vi "LabVIEW_ArduinoControls.vi"() -> ()   [LabVIEW 2020]
uses:
  <vilib>/Instr/_visa.llb/VISA Configure Serial Port (Instr).vi
panel:
  in  "DRILL STOP":bool
  in  "Drill Speed Arduino 2 Write Stop":bool
  in  "Slow Down":bool
  in  "Speed Up":bool
  in  "Drill Speed Arduino 2 Write":refnum<visa-resource-name>
  in  "Stepper Arduino 1 Serial Read":refnum<visa-resource-name>
  out "Weight on Bit A1":dbl[](graph)
  out "Vertical Motor Speed A1":dbl[](graph)
  out "Data Packet Arduini 1 Matched":i32
  in  "Arduino 1 Read Stop 2":bool
  in  "Arduino 1 Read Stop":bool
  in  "Emergency Stop! 3":bool
  in  "Emergency Stop! 2":bool
  in  "GO DOWN 3":bool
  in  "GO DOWN 2":bool
  in  "GO UP 3":bool
  in  "GO UP 2":bool
  in  "MAX SPEED 3":bool
  in  "MAX SPEED 2":bool
  in  "SLOWEST SPEED 3":bool
  in  "SLOWEST SPEED 2":bool
  in  "Decellerate 3":bool
  in  "Decellerate 2":bool
  in  "Accelerate 3":bool
  in  "Accelerate 2":bool
  in  "Drill Speed Arduino 2 Serial Read":refnum<visa-resource-name>
  out "Data Packet Received":i32
  out "Drill Amps A2":dbl[](graph)
  in  "GO UP":bool
  in  "GO DOWN":bool
  in  "MAX SPEED":bool
  in  "SLOWEST SPEED":bool
  out "System Amps A2":dbl[](graph)
  out "concatenated string":string
  in  "Arduino 2 Write Stop":bool
  in  "Emergency Stop!":bool
  in  "Decellerate":bool
  in  "Stepper Arduino 1 Write":refnum<visa-resource-name>
  in  "Accelerate":bool
  # "WINCH CONTROLS"
  # "VERTICAL STEPPER MOTOR CONTROLS"
  # "HORIZONTAL STEPPER MOTOR CONTROLS"
  # "Drill Speed Controls"
  # "-1 Means Not Found\nany value greater than 0 corresponds to the amount\nof matching characters found"
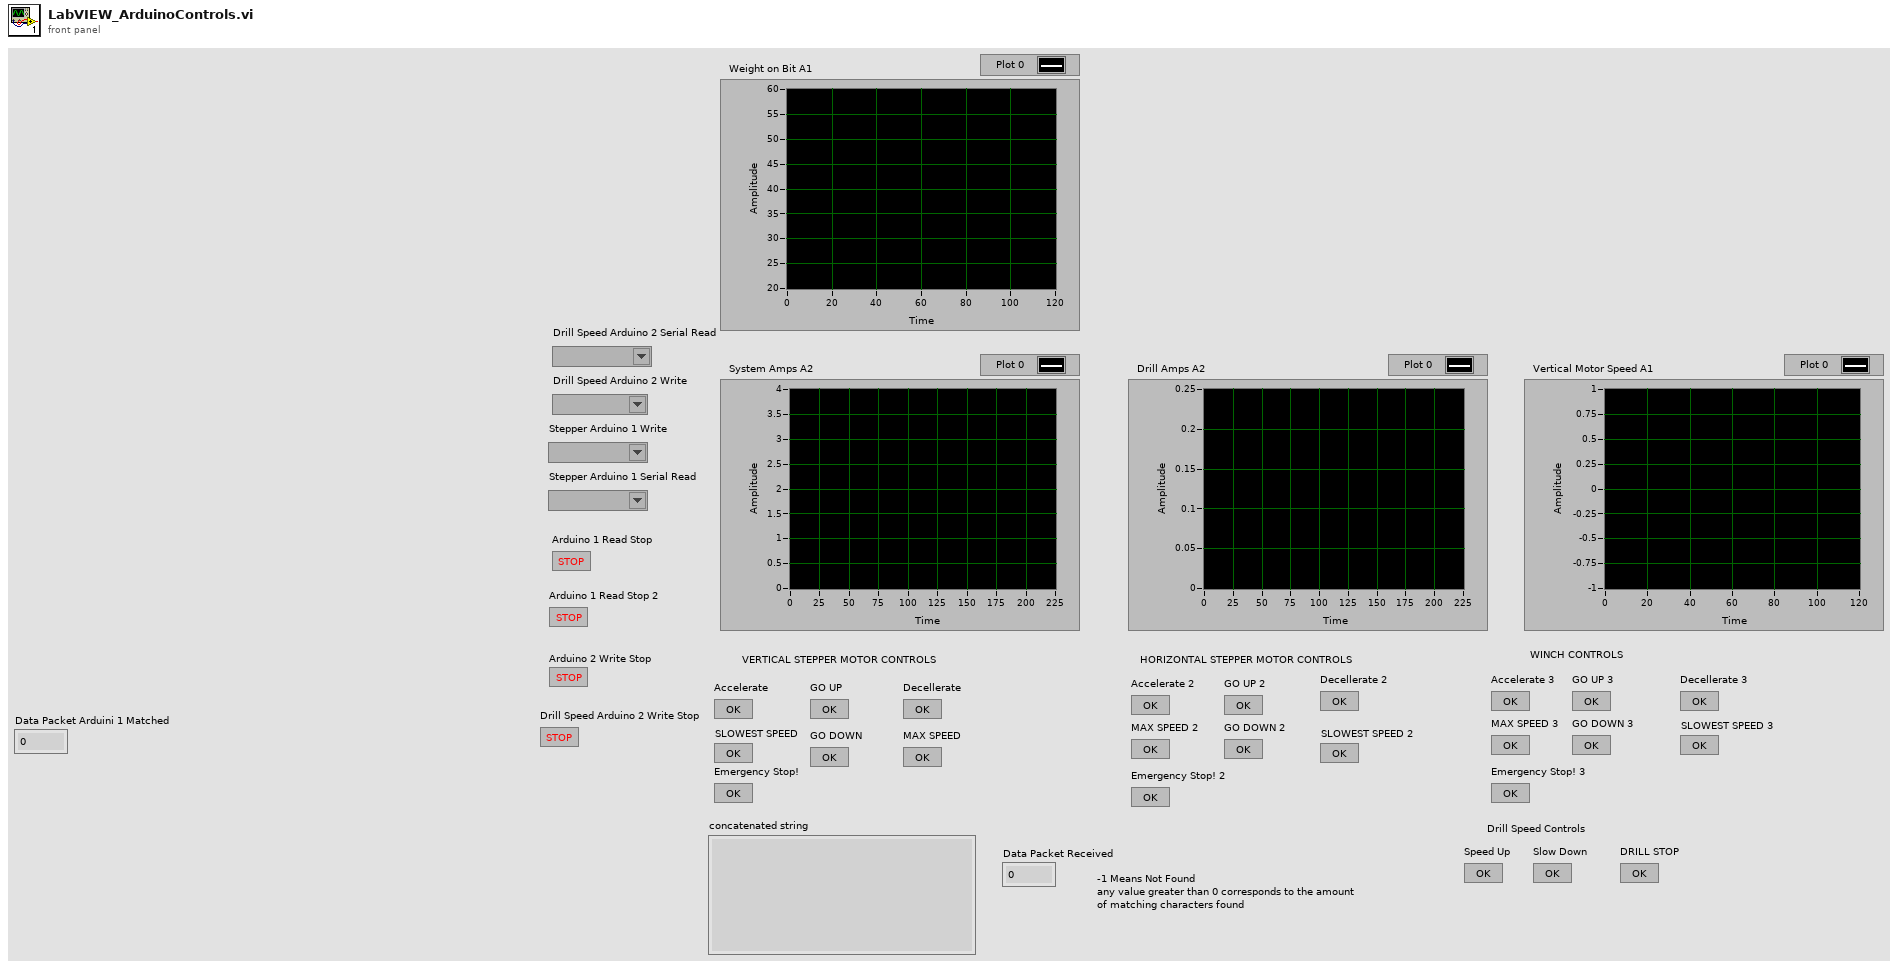
[diagram p1: front panel]
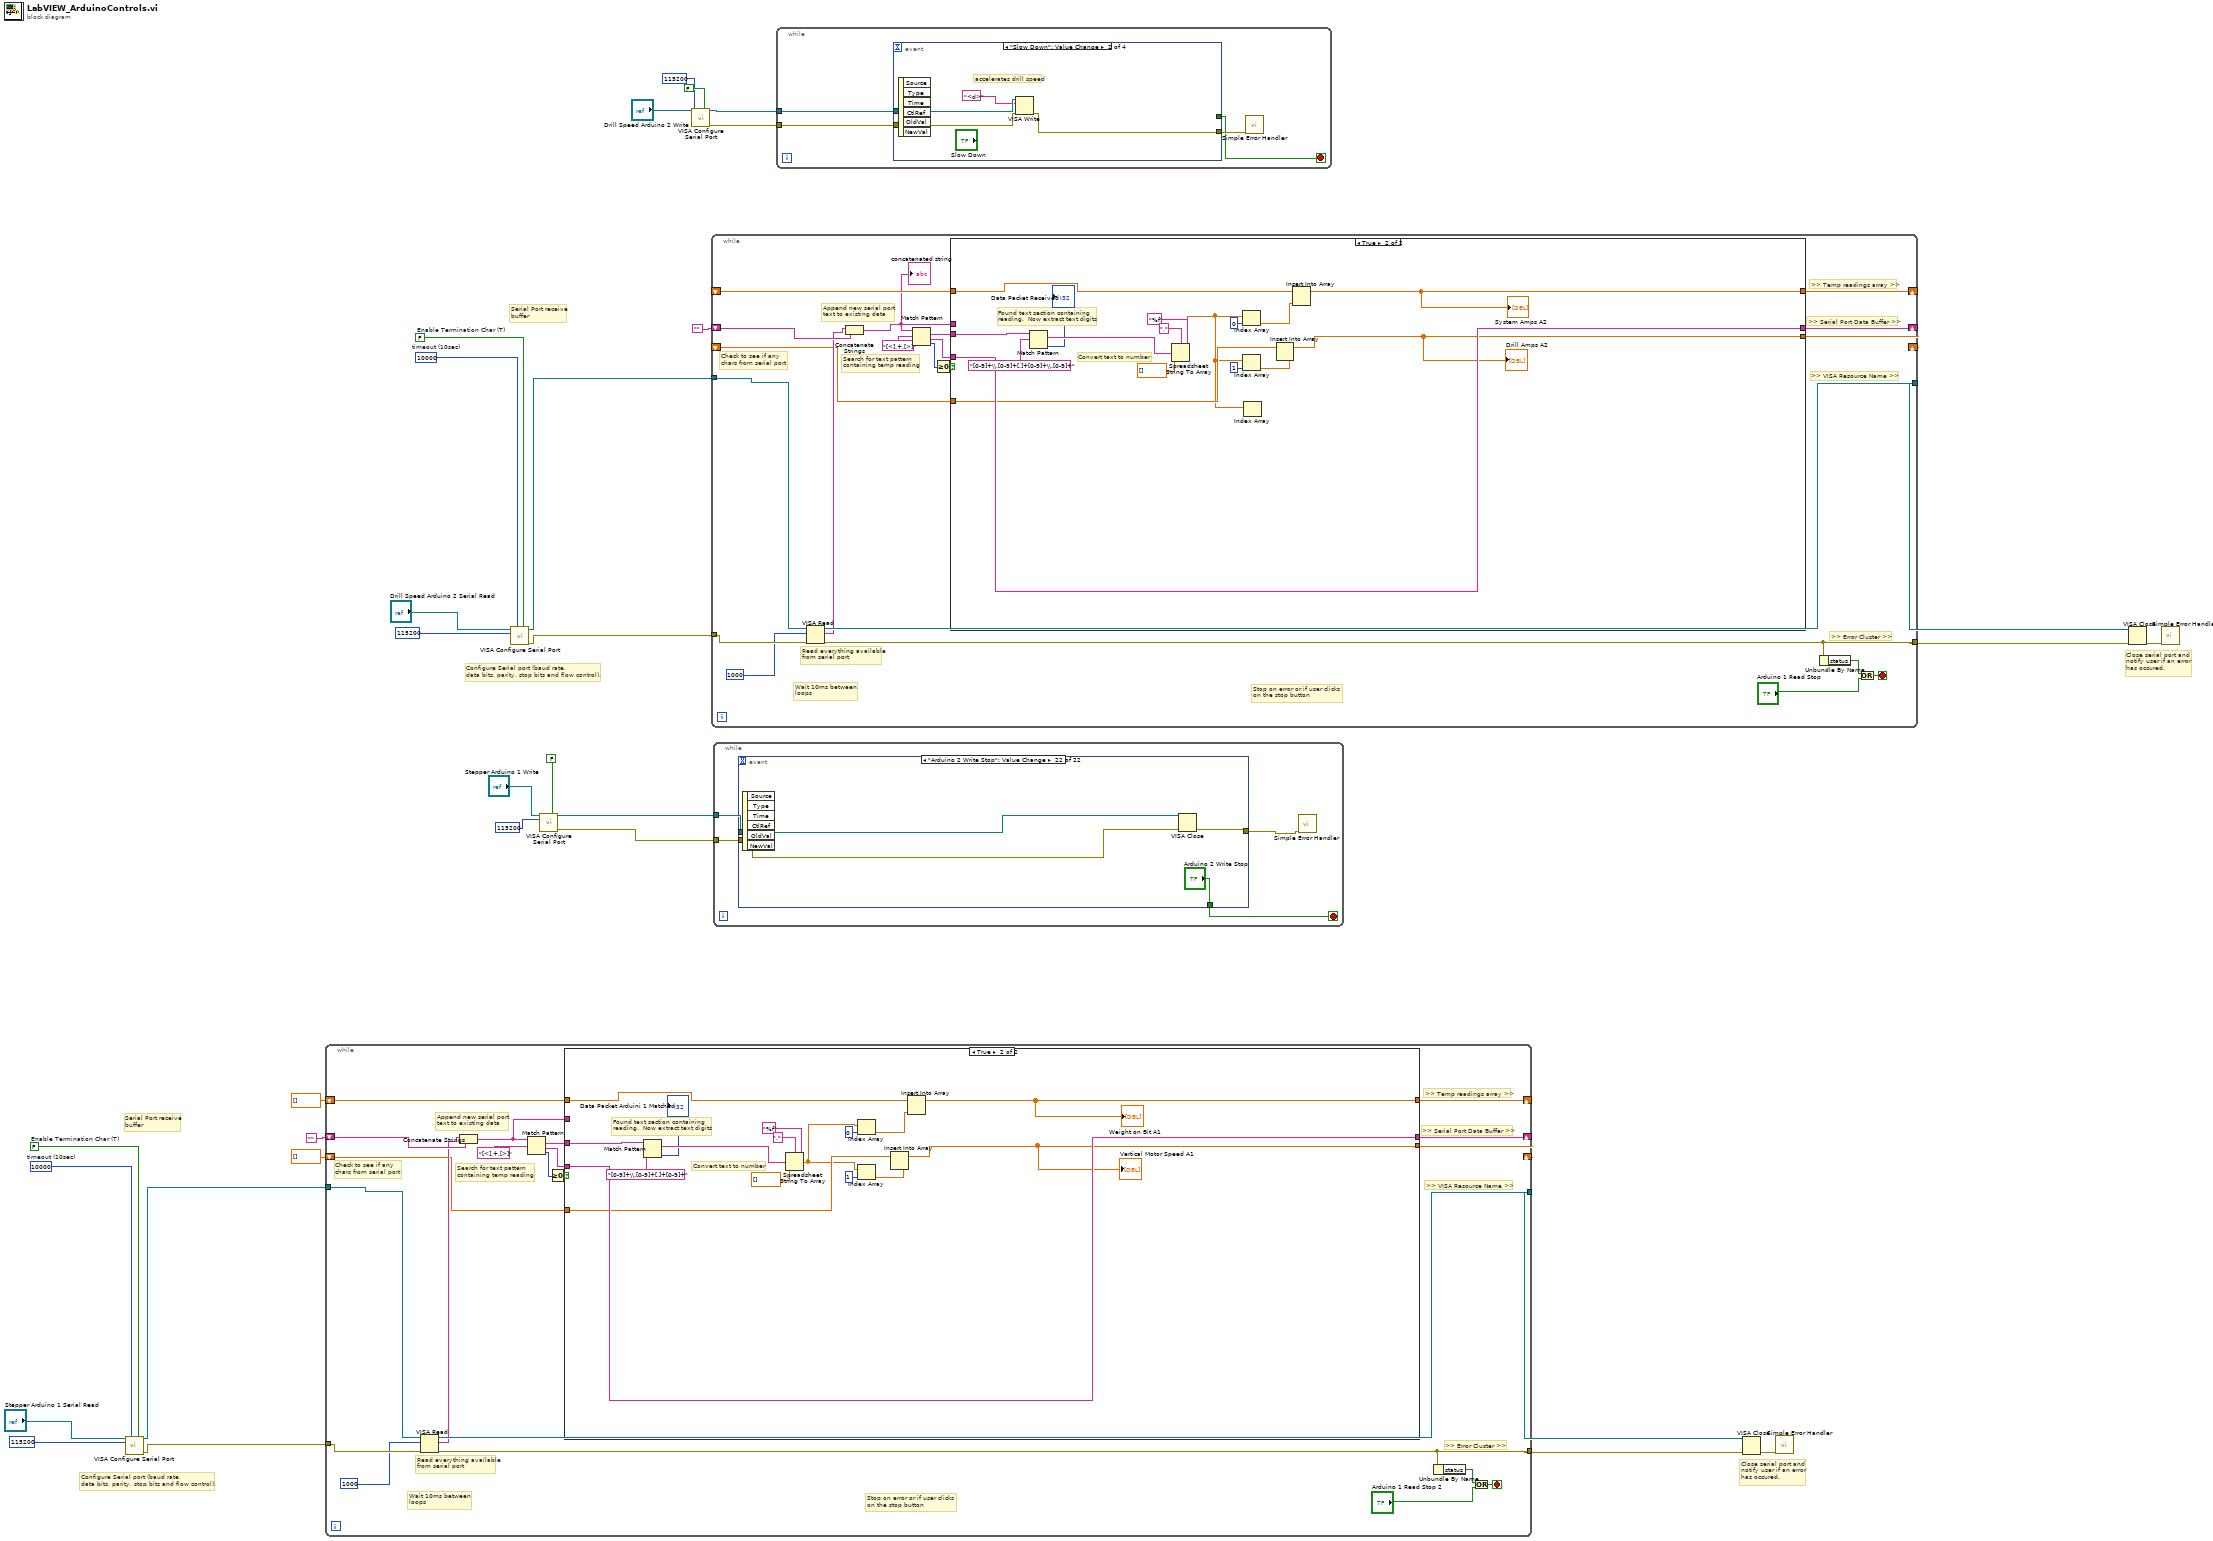
[diagram p0: block diagram]
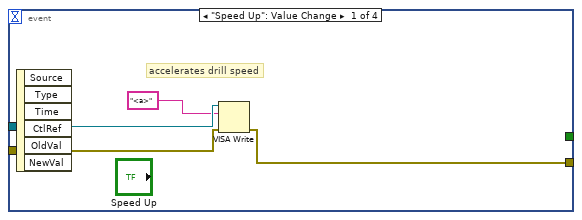
[diagram p2: hidden frame]
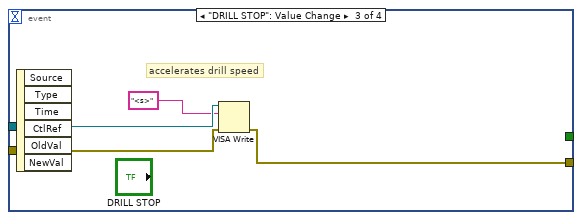
[diagram p3: hidden frame]
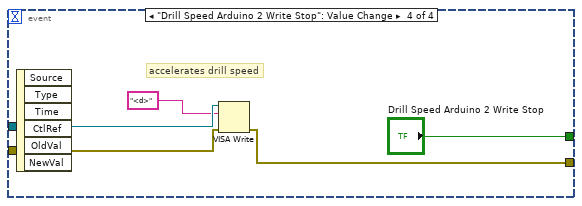
[diagram p4: hidden frame]
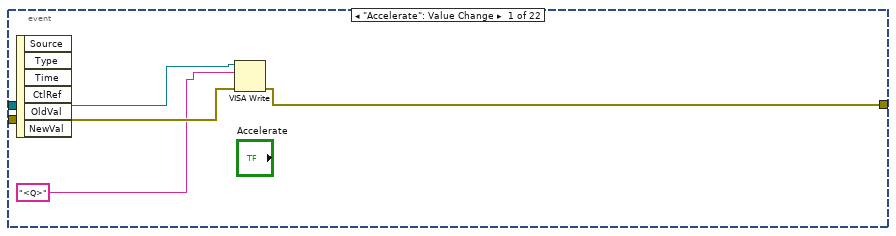
[diagram p7: hidden frame]
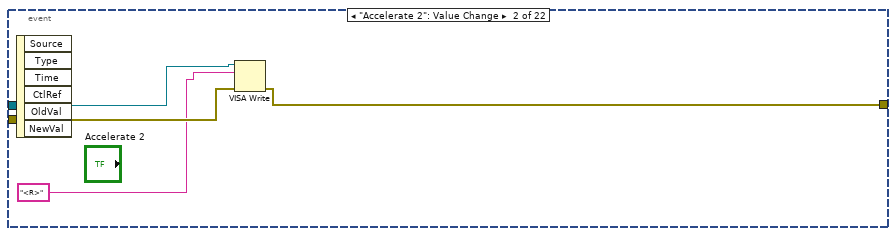
[diagram p8: hidden frame]
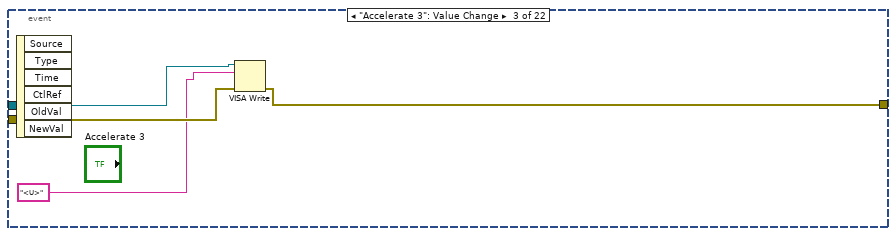
[diagram p9: hidden frame]
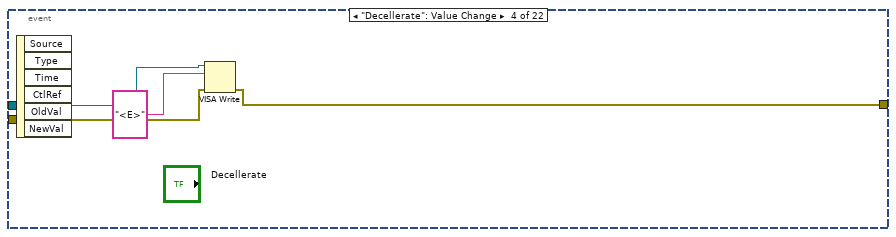
[diagram p10: hidden frame]
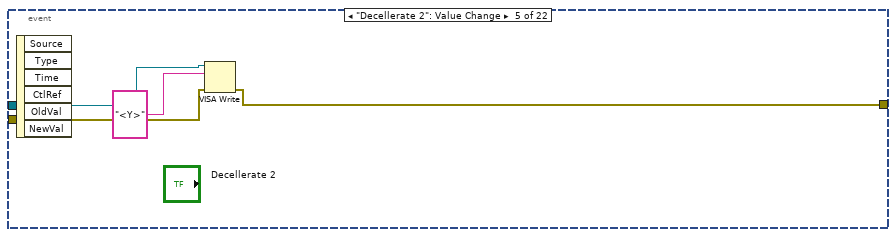
[diagram p11: hidden frame]
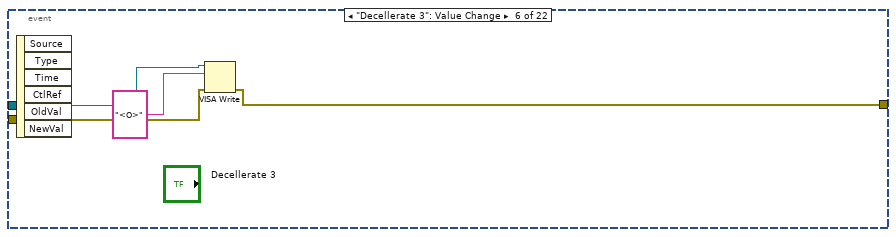
[diagram p12: hidden frame]
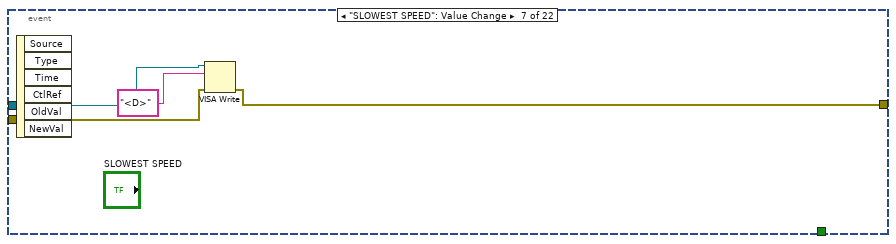
[diagram p13: hidden frame]
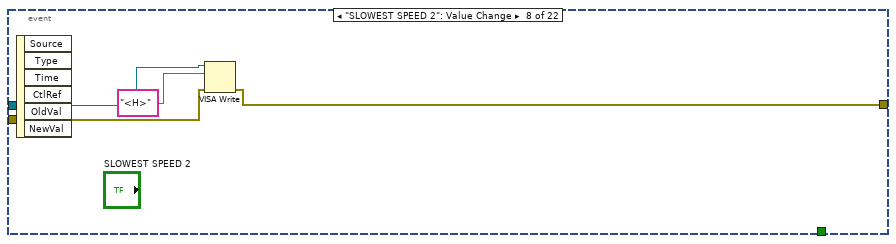
[diagram p14: hidden frame]
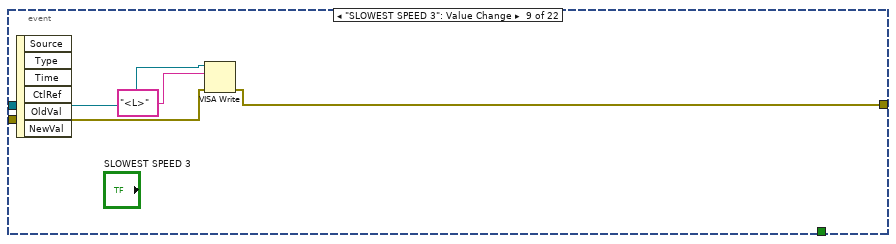
[diagram p15: hidden frame]
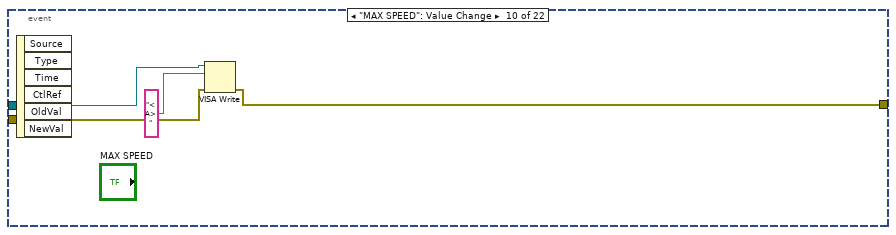
[diagram p16: hidden frame]
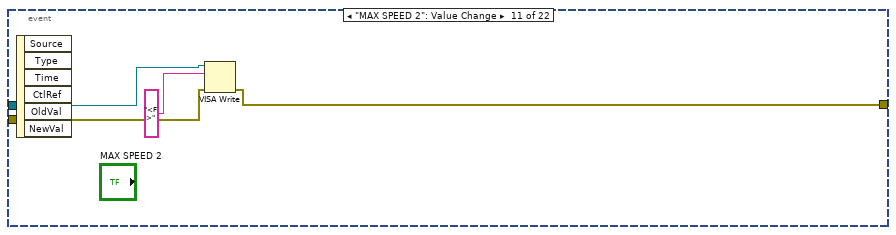
[diagram p17: hidden frame]
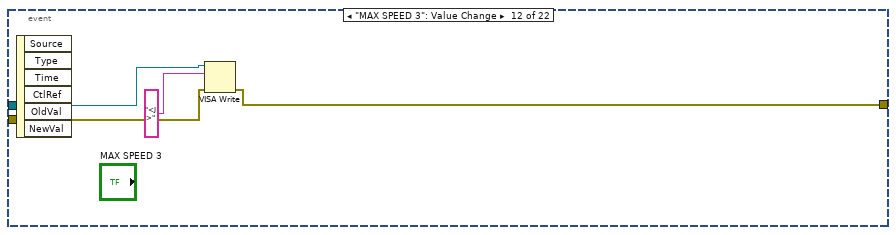
[diagram p18: hidden frame]
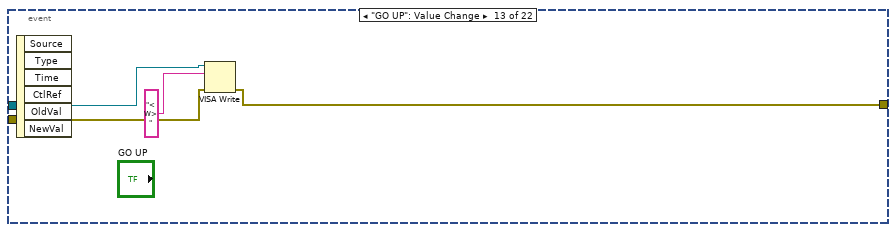
[diagram p19: hidden frame]
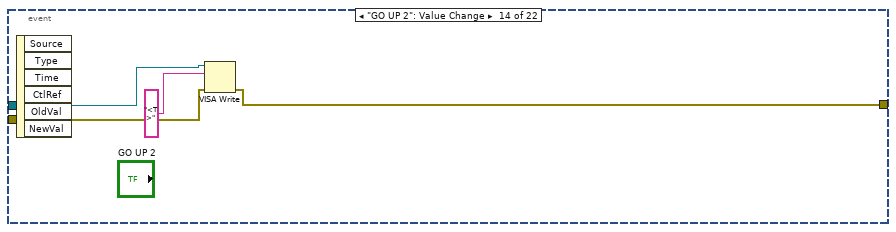
[diagram p20: hidden frame]
diagram:
  w13 = FALSE  # Enable Termination Char (T)
  w14 = u32 10000  # timeout (10sec)
  w24 = FALSE  # Enable Termination Char (T)
  w25 = u32 10000  # timeout (10sec)
  # "Close serial port and\nnotify user if an error\nhas occured."
  # "Serial Port receive\nbuffer"
  # "Configure Serial port (baud rate,\ndata bits, parity, stop bits and flow control)."
  # "Close serial port and\nnotify user if an error\nhas occured."
  # "Serial Port receive\nbuffer"
  # "Configure Serial port (baud rate,\ndata bits, parity, stop bits and flow control)."
  n1 = call-poly "VISA Configure Serial Port"("VISA resource name"="Stepper Arduino 1 Serial Read", "timeout (10sec)"=w14, "Enable Termination\nChar (T)"=w13, "baud rate (9600)"=u32 115200) -> ("VISA resource name out"=w10:refnum<visa-resource-name>, "error out"=w9:errorcluster)  [unwired: 10 in]
  n2 = while {
    tunnel: [w51] -> w17
    tunnel: [w53] -> w16
    shift-right: [w46] -> _
    shift-left: "" -> [w52]
    shift-right: [w48] -> _
    shift-left: dbl[] [] -> [w47]
    tunnel: w10 -> [w45]
    tunnel: w9 -> [w44]
    shift-right: [w36] -> _
    shift-left: dbl[] [] -> [w35]
    stop <- w50 stop-if-true
    # "Search for text pattern\ncontaining temp reading"
    # "Append new serial port\ntext to existing data"
    # "Read everything available\nfrom serial port"
    # "Wait 10ms between \nloops"
    # "Stop on error or if user clicks \non the stop button"
    # ">> Error Cluster >>"
    # ">> VISA Resource Name >>"
    # ">> Temp readings array >>"
    # ">> Serial Port Data Buffer >>"
    # "Check to see if any\nchars from serial port"
    n3 = VISA Read(VISA resource name=w45, byte count=u32 1000, error in (no error)=w44) -> (VISA resource name out=w53:refnum<visa-resource-name>, read buffer=w38:string, error out=w51:errorcluster)  [unwired: 1 out]
    n4 = Concatenate Strings(w38, w52) -> (w33:string)
    n5 = Match Pattern(string=w33, regular expression="[<].+.[>]") -> (match substring=w40:string, after substring=w39:string, offset past match=w42:i32)  [unwired: 1 in, 1 out]
    n6 = Greater Or Equal To 0?(x=w42) -> (x >= 0?=w41:bool)
    n7 = case shown="True" w41 {
      tunnel: w40 -> [_ w72]
      tunnel: w39 -> [_ w73]
      tunnel: [w54 w73] -> w46
      tunnel: [w56 w70] -> w48
      tunnel: w47 -> [w56 w58]
      tunnel: [w55 w61] -> w36
      tunnel: w35 -> [w55 w62]
      tunnel: w33 -> [w54 _]
      frame False {
        # "Did not find text pattern in the buffer.  Try again in the next loop after new data \nhas been received."
      }
      frame True {
        # "Convert text to number"
        # "Found text section containing \nreading.  Now extract text digits"
        n8 = Match Pattern(string=w72, regular expression="[0-9]+\\.[0-9]+[,]+[0-9]+") -> (match substring=w65:string, offset past match=→"Data Packet Arduini 1 Matched":i32)  [unwired: 1 in, 2 out]
        n9 = Spreadsheet String To Array(delimiter (Tab)=",", format string="%f", spreadsheet string=w65, array type (2D Dbl)=dbl[] []) -> (array=w57:dbl[])
        n10 = Index Array(array=w57, index=0 ("index (row)")) -> (element=w64:dbl)
        n11 = Index Array(array=w57, index=1 ("index (row)")) -> (element=w63:dbl)
        n12 = Insert Into Array(array=w62, new element=w63) -> (w61:dbl[])  [unwired: 1 in]
        "Vertical Motor Speed A1" <- w61
        n13 = Insert Into Array(array=w58, new element=w64) -> (w70:dbl[])  [unwired: 1 in]
        "Weight on Bit A1" <- w70
      }
    }
    n14 = Unbundle By Name(w51) -> ("status"=w49:bool)
    n15 = Or(x=w49, y="Arduino 1 Read Stop 2") -> (x .or. y?=w50:bool)
  }
  n16 = call-poly "VISA Configure Serial Port"("VISA resource name"="Drill Speed Arduino 2 Serial Read", "timeout (10sec)"=w25, "Enable Termination\nChar (T)"=w24, "baud rate (9600)"=u32 115200) -> ("VISA resource name out"=w21:refnum<visa-resource-name>, "error out"=w20:errorcluster)  [unwired: 10 in]
  n17 = call-poly "VISA Configure Serial Port"("VISA resource name"="Stepper Arduino 1 Write", "Enable Termination\nChar (T)"=FALSE ("Enable Termination\nChar (T)"), "baud rate (9600)"=u32 115200) -> ("VISA resource name out"=w32:refnum<visa-resource-name>, "error out"=w31:errorcluster)  [unwired: 11 in]
  n18 = call-poly "VISA Configure Serial Port"("VISA resource name"="Drill Speed Arduino 2 Write", "Enable Termination\nChar (T)"=FALSE ("Enable Termination\nChar (T)"), "baud rate (9600)"=u32 115200) -> ("VISA resource name out"=w7:refnum<visa-resource-name>, "error out"=w6:errorcluster)  [unwired: 11 in]
  n19 = while {
    tunnel: [w92] -> w28
    tunnel: [w94] -> w27
    shift-right: [w87] -> _
    shift-left: "" -> [w93]
    shift-right: [w89] -> _
    shift-left: _ -> [w88]
    tunnel: w21 -> [w86]
    tunnel: w20 -> [w85]
    shift-right: [w77] -> _
    shift-left: _ -> [w76]
    stop <- w91 stop-if-true
    # "Search for text pattern\ncontaining temp reading"
    # "Append new serial port\ntext to existing data"
    # "Read everything available\nfrom serial port"
    # "Wait 10ms between \nloops"
    # "Stop on error or if user clicks \non the stop button"
    # ">> Error Cluster >>"
    # ">> VISA Resource Name >>"
    # ">> Temp readings array >>"
    # ">> Serial Port Data Buffer >>"
    # "Check to see if any\nchars from serial port"
    n20 = VISA Read(VISA resource name=w86, byte count=u32 1000, error in (no error)=w85) -> (VISA resource name out=w94:refnum<visa-resource-name>, read buffer=w79:string, error out=w92:errorcluster)  [unwired: 1 out]
    n21 = Concatenate Strings(w79, w93) -> (w74:string)
    "concatenated string" <- w74
    n22 = Match Pattern(string=w74, regular expression="[<].+.[>]") -> (match substring=w81:string, after substring=w80:string, offset past match=w83:i32)  [unwired: 1 in, 1 out]
    n23 = Greater Or Equal To 0?(x=w83) -> (x >= 0?=w82:bool)
    n24 = case shown="True" w82 {
      tunnel: w81 -> [_ w113]
      tunnel: w80 -> [_ w114]
      tunnel: [w95 w114] -> w87
      tunnel: [w97 w111] -> w89
      tunnel: w88 -> [w97 w99]
      tunnel: [w96 w102] -> w77
      tunnel: w76 -> [w96 w103]
      tunnel: w74 -> [w95 _]
      frame False {
        # "Did not find text pattern in the buffer.  Try again in the next loop after new data \nhas been received."
      }
      frame True {
        # "Convert text to number"
        # "Found text section containing \nreading.  Now extract text digits"
        n25 = Match Pattern(string=w113, regular expression="[0-9]+\\.[0-9]+[,]+[0-9]+\\.[0-9]+") -> (match substring=w106:string, offset past match=→"Data Packet Received":i32)  [unwired: 1 in, 2 out]
        n26 = Spreadsheet String To Array(delimiter (Tab)=",", format string="%f", spreadsheet string=w106, array type (2D Dbl)=dbl[] []) -> (array=w98:dbl[])
        n27 = Index Array(array=w98, index=0 ("index (row)")) -> (element=w105:dbl)
        n28 = Index Array(array=w98, index=1 ("index (row)")) -> (element=w104:dbl)
        n29 = Index Array(array=w98) -> ()  [unwired: 1 in, 1 out]
        n30 = Insert Into Array(array=w103, new element=w104) -> (w102:dbl[])  [unwired: 1 in]
        "Drill Amps A2" <- w102
        n31 = Insert Into Array(array=w99, new element=w105) -> (w111:dbl[])  [unwired: 1 in]
        "System Amps A2" <- w111
      }
    }
    n32 = Unbundle By Name(w92) -> ("status"=w90:bool)
    n33 = Or(x=w90, y="Arduino 1 Read Stop") -> (x .or. y?=w91:bool)
  }
  n34 = while {
    tunnel: w32 -> [w118]
    tunnel: w31 -> [w117]
    stop <- w115 stop-if-true
    n35 = event shown="[21] \"Arduino 2 Write Stop\": Value Change" {
      selector: _ -> [_ _ _ _ _ _ _ _ _ _ _ _ _ _ _ _ _ _ _ _ _ _]
      dyn-events: _ -> [_ _ _ _ _ _ _ _ _ _ _ _ _ _ _ _ _ _ _ _ _ _]
      timeout: _ -> [_ _ _ _ _ _ _ _ _ _ _ _ _ _ _ _ _ _ _ _ _ _]
      tunnel: [w122 w126 w130 w134 w138 w142 w146 w150 w154 w158 w162 w166 w170 w174 w178 w182 w186 w190 w194 w198 w202 w206] -> w116
      tunnel: w118 -> [w121 w125 w129 w132 w136 w140 w144 w148 w152 w156 w160 w164 w168 w172 w176 w180 w184 w188 w192 w196 w200 w205]
      tunnel: w117 -> [w120 w124 w128 w131 w135 w139 w143 w147 w151 w155 w159 w163 w167 w171 w175 w179 w183 w187 w191 w195 w199 w204]
      tunnel: [_ _ _ _ _ _ _ _ _ _ _ _ _ _ _ _ _ _ _ _ _ "Arduino 2 Write Stop"] -> w115
      event "Accelerate": Value Change {
        n36 = event-data() -> ()  [unwired: 1 in, 6 out]
        n37 = VISA Write(VISA resource name=w121, write buffer="<Q>", error in (no error)=w120) -> (error out=w122:errorcluster)  [unwired: 2 out]
      }
      event "Accelerate 2": Value Change {
        n38 = event-data() -> ()  [unwired: 1 in, 6 out]
        n39 = VISA Write(VISA resource name=w125, write buffer="<R>", error in (no error)=w124) -> (error out=w126:errorcluster)  [unwired: 2 out]
      }
      event "Accelerate 3": Value Change {
        n40 = event-data() -> ()  [unwired: 1 in, 6 out]
        n41 = VISA Write(VISA resource name=w129, write buffer="<U>", error in (no error)=w128) -> (error out=w130:errorcluster)  [unwired: 2 out]
      }
      event "Decellerate": Value Change {
        n42 = event-data() -> ()  [unwired: 1 in, 6 out]
        n43 = VISA Write(VISA resource name=w132, write buffer="<E>", error in (no error)=w131) -> (error out=w134:errorcluster)  [unwired: 2 out]
      }
      event "Decellerate 2": Value Change {
        n44 = event-data() -> ()  [unwired: 1 in, 6 out]
        n45 = VISA Write(VISA resource name=w136, write buffer="<Y>", error in (no error)=w135) -> (error out=w138:errorcluster)  [unwired: 2 out]
      }
      event "Decellerate 3": Value Change {
        n46 = event-data() -> ()  [unwired: 1 in, 6 out]
        n47 = VISA Write(VISA resource name=w140, write buffer="<O>", error in (no error)=w139) -> (error out=w142:errorcluster)  [unwired: 2 out]
      }
      event "SLOWEST SPEED": Value Change {
        n48 = event-data() -> ()  [unwired: 1 in, 6 out]
        n49 = VISA Write(VISA resource name=w144, write buffer="<D>", error in (no error)=w143) -> (error out=w146:errorcluster)  [unwired: 2 out]
      }
      event "SLOWEST SPEED 2": Value Change {
        n50 = event-data() -> ()  [unwired: 1 in, 6 out]
        n51 = VISA Write(VISA resource name=w148, write buffer="<H>", error in (no error)=w147) -> (error out=w150:errorcluster)  [unwired: 2 out]
      }
      event "SLOWEST SPEED 3": Value Change {
        n52 = event-data() -> ()  [unwired: 1 in, 6 out]
        n53 = VISA Write(VISA resource name=w152, write buffer="<L>", error in (no error)=w151) -> (error out=w154:errorcluster)  [unwired: 2 out]
      }
      event "MAX SPEED": Value Change {
        n54 = event-data() -> ()  [unwired: 1 in, 6 out]
        n55 = VISA Write(VISA resource name=w156, write buffer="<A>", error in (no error)=w155) -> (error out=w158:errorcluster)  [unwired: 2 out]
      }
      event "MAX SPEED 2": Value Change {
        n56 = event-data() -> ()  [unwired: 1 in, 6 out]
        n57 = VISA Write(VISA resource name=w160, write buffer="<F>", error in (no error)=w159) -> (error out=w162:errorcluster)  [unwired: 2 out]
      }
      event "MAX SPEED 3": Value Change {
        n58 = event-data() -> ()  [unwired: 1 in, 6 out]
        n59 = VISA Write(VISA resource name=w164, write buffer="<J>", error in (no error)=w163) -> (error out=w166:errorcluster)  [unwired: 2 out]
      }
      event "GO UP": Value Change {
        n60 = event-data() -> ()  [unwired: 1 in, 6 out]
        n61 = VISA Write(VISA resource name=w168, write buffer="<W>", error in (no error)=w167) -> (error out=w170:errorcluster)  [unwired: 2 out]
      }
      event "GO UP 2": Value Change {
        n62 = event-data() -> ()  [unwired: 1 in, 6 out]
        n63 = VISA Write(VISA resource name=w172, write buffer="<T>", error in (no error)=w171) -> (error out=w174:errorcluster)  [unwired: 2 out]
      }
      event "GO UP 3": Value Change {
        n64 = event-data() -> ()  [unwired: 1 in, 6 out]
        n65 = VISA Write(VISA resource name=w176, write buffer="<I>", error in (no error)=w175) -> (error out=w178:errorcluster)  [unwired: 2 out]
      }
      event "GO DOWN": Value Change {
        n66 = event-data() -> ()  [unwired: 1 in, 6 out]
        n67 = VISA Write(VISA resource name=w180, write buffer="<S>", error in (no error)=w179) -> (error out=w182:errorcluster)  [unwired: 2 out]
      }
      event "GO DOWN 2": Value Change {
        n68 = event-data() -> ()  [unwired: 1 in, 6 out]
        n69 = VISA Write(VISA resource name=w184, write buffer="<G>", error in (no error)=w183) -> (error out=w186:errorcluster)  [unwired: 2 out]
      }
      event "GO DOWN 3": Value Change {
        n70 = event-data() -> ()  [unwired: 1 in, 6 out]
        n71 = VISA Write(VISA resource name=w188, write buffer="<K>", error in (no error)=w187) -> (error out=w190:errorcluster)  [unwired: 2 out]
      }
      event "Emergency Stop!": Value Change {
        n72 = event-data() -> ()  [unwired: 1 in, 6 out]
        n73 = VISA Write(VISA resource name=w192, write buffer="<Z>", error in (no error)=w191) -> (error out=w194:errorcluster)  [unwired: 2 out]
      }
      event "Emergency Stop! 2": Value Change {
        n74 = event-data() -> ()  [unwired: 1 in, 6 out]
        n75 = VISA Write(VISA resource name=w196, write buffer="<C>", error in (no error)=w195) -> (error out=w198:errorcluster)  [unwired: 2 out]
      }
      event "Emergency Stop! 3": Value Change {
        n76 = event-data() -> ()  [unwired: 1 in, 6 out]
        n77 = VISA Write(VISA resource name=w200, write buffer="<N>", error in (no error)=w199) -> (error out=w202:errorcluster)  [unwired: 2 out]
      }
      event "Arduino 2 Write Stop": Value Change {
        n78 = event-data() -> ()  [unwired: 1 in, 6 out]
        n79 = VISA Close(VISA resource name=w205, error in (no error)=w204) -> (error out=w206:errorcluster)
      }
    }
    n80 = call <vilib>:"Simple Error Handler.vi"("error in (no error)"=w116) -> ()  [unwired: 4 in, 5 out]
  }
  n81 = while {
    tunnel: w7 -> [w210]
    tunnel: w6 -> [w209]
    stop <- w207 stop-if-true
    n82 = event shown="[1] \"Slow Down\": Value Change" {
      selector: _ -> [_ _ _ _]
      dyn-events: _ -> [_ _ _ _]
      timeout: _ -> [_ _ _ _]
      tunnel: w210 -> [w214 w218 w222 w227]
      tunnel: w209 -> [w213 w217 w221 w226]
      tunnel: [w211 w215 w219 w224] -> w208
      tunnel: [_ _ _ "Drill Speed Arduino 2 Write Stop"] -> w207
      event "Speed Up": Value Change {
        # "accelerates drill speed"
        n83 = event-data() -> ()  [unwired: 1 in, 6 out]
        n84 = VISA Write(VISA resource name=w214, write buffer="<a>", error in (no error)=w213) -> (error out=w211:errorcluster)  [unwired: 2 out]
      }
      event "Slow Down": Value Change {
        # "accelerates drill speed"
        n85 = event-data() -> ()  [unwired: 1 in, 6 out]
        n86 = VISA Write(VISA resource name=w218, write buffer="<d>", error in (no error)=w217) -> (error out=w215:errorcluster)  [unwired: 2 out]
      }
      event "DRILL STOP": Value Change {
        # "accelerates drill speed"
        n87 = event-data() -> ()  [unwired: 1 in, 6 out]
        n88 = VISA Write(VISA resource name=w222, write buffer="<s>", error in (no error)=w221) -> (error out=w219:errorcluster)  [unwired: 2 out]
      }
      event "Drill Speed Arduino 2 Write Stop": Value Change {
        # "accelerates drill speed"
        n89 = event-data() -> ()  [unwired: 1 in, 6 out]
        n90 = VISA Write(VISA resource name=w227, write buffer="<d>", error in (no error)=w226) -> (error out=w224:errorcluster)  [unwired: 2 out]
      }
    }
    n91 = call <vilib>:"Simple Error Handler.vi"("error in (no error)"=w208) -> ()  [unwired: 4 in, 5 out]
  }
  n92 = VISA Close(VISA resource name=w16, error in (no error)=w17) -> (error out=w15:errorcluster)
  n93 = call <vilib>:"Simple Error Handler.vi"("error in (no error)"=w15) -> ()  [unwired: 4 in, 5 out]
  n94 = VISA Close(VISA resource name=w27, error in (no error)=w28) -> (error out=w26:errorcluster)
  n95 = call <vilib>:"Simple Error Handler.vi"("error in (no error)"=w26) -> ()  [unwired: 4 in, 5 out]
